vi "Move To Raw Relative.vi"(6 "Rotation Angle":dbl, 7 "Wait?":bool=TRUE, 8 "error in":errorcluster, 9 "Speed(mm/s)":dbl=5.0, 10 "Delta":refnum<class "Vec3d.lvclass">, 11 "Gantry in":refnum<class "Gantry.lvclass">) -> (0 "error out":errorcluster, 3 "Gantry out":refnum<class "Gantry.lvclass">)   [LabVIEW 2026, in "Gantry.lvclass"]
uses:
  Gantry.lvclass
  Vec3d Class/Vec3d.lvclass
  Gantry.lvclass/Gantry.ctl
  <instrlib>/Aerotech Automation1/Commands/Motion/typedefs/MoveLinear parameters.ctl
  <instrlib>/Aerotech Automation1/Aerotech Automation1.lvlib
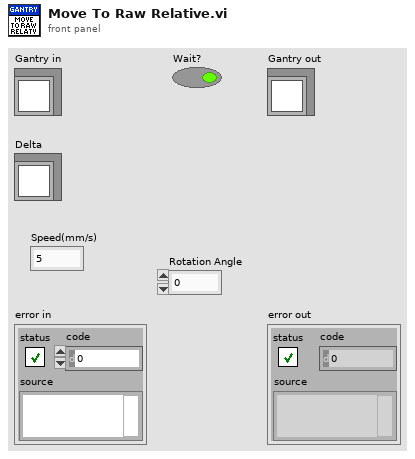
[diagram p1: front panel]
types:
  T1 = typedef "Aerotech Automation1.lvlib/MoveLinear parameters.ctl" = cluster{"coordinatedSpeed":dbl, "distances":dbl[], "axes":string[]}
  T2 = typedef "Virtual Modes.ctl" = enum16{"Nonvirtual", "Virtual"}
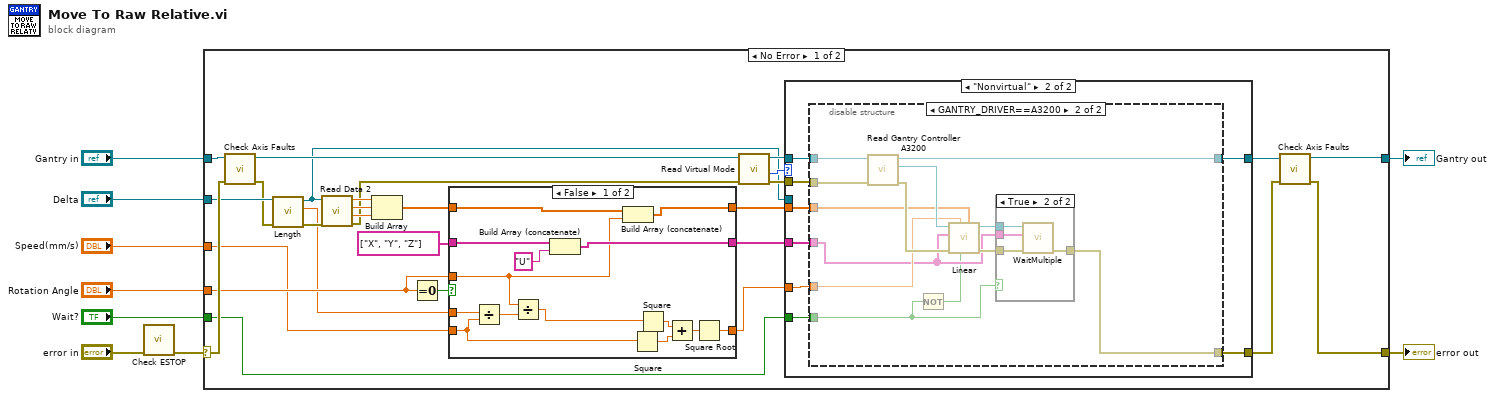
[diagram p0: block diagram]
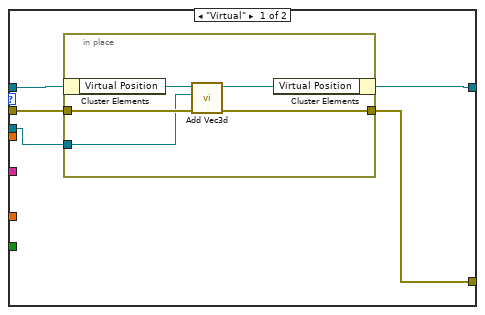
[diagram p3: hidden frame]
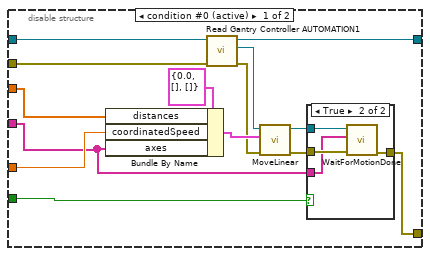
[diagram p4: hidden frame]
diagram:
  n1 = call "Check ESTOP.vi"("error in"="error in") -> ("error out"=w3:errorcluster)  [unwired: 10 in]
  n2 = case shown="No Error" w3 {
    selector: w3 -> [w33 w111]
    tunnel: [w11 w111] -> w8
    tunnel: [w10 w110] -> w7
    tunnel: "Gantry in" -> [w35 w110]
    tunnel: "Speed(mm/s)" -> [w20 _]
    tunnel: "Delta" -> [w18 _]
    tunnel: "Wait?" -> [w28 _]
    tunnel: "Rotation Angle" -> [w24 _]
    frame No Error {
      n3 = call "Check Axis Faults.vi"("error in (no error)"=w33, "Gantry in"=w35) -> ("error out"=w16:errorcluster, "Gantry out"=w34:refnum<class "Gantry.lvclass">)  [unwired: 8 in]
      n4 = call-dynamic "Length.vi"("error in"=w16, "Vec3d in"=w18) -> ("error out"=w15:errorcluster, "Length"=w14:dbl, "Vec3d out"=w17:refnum<class "Vec3d.lvclass">)  [unwired: 7 in]
      n5 = call-dynamic "Read Data 2.vi"("error in"=w15, "Vec3d in"=w17) -> ("error out"=w29:errorcluster, "Z"=w30:dbl, "Y"=w31:dbl, "X"=w32:dbl)  [unwired: 6 in]
      n6 = Build Array(w32, w31, w30) -> (w27:dbl[])
      n7 = Equal To 0?(x=w24) -> (x = 0?=w25:bool)
      n8 = case shown="False" w25 {
        tunnel: w24 -> [w38 _]
        tunnel: w27 -> [w41 w53]
        tunnel: string[] ["X", "Y", "Z"] -> [w43 w52]
        tunnel: w20 -> [w46 w54]
        tunnel: [w48 w54] -> w19
        tunnel: [w40 w53] -> w22
        tunnel: [w39 w52] -> w21
        tunnel: w14 -> [w47 _]
        frame False {
          n9 = Divide(x=w47, y=w46) -> (x/y=w45:dbl)
          n10 = Divide(x=w38, y=w45) -> (x/y=w44:dbl)
          n11 = Build Array (concatenate)(w43, "U") -> (w39:string[])
          n12 = Build Array (concatenate)(w41, w38) -> (w40:dbl[])
          n13 = Square(x=w46) -> (x^2=w51:dbl)
          n14 = Square(x=w44) -> (x^2=w50:dbl)
          n15 = Add(x=w50, y=w51) -> (x+y=w49:dbl)
          n16 = Square Root(x=w49) -> (sqrt(x)=w48:dbl)
        }
        frame True {
        }
      }
      n17 = call-dynamic "Read Virtual Mode.vi"("error in (no error)"=w29, "Gantry in"=w34) -> ("error out"=w23:errorcluster, "Virtual Mode"=w36:T2, "Gantry out"=w37:refnum<class "Gantry.lvclass">)  [unwired: 6 in, 1 out]
      n18 = case shown="\"Nonvirtual\"" w36 {
        tunnel: w28 -> [_ w70]
        tunnel: [w56 w65] -> w12
        tunnel: [w58 w66] -> w13
        tunnel: w37 -> [w59 w72]
        tunnel: w17 -> [w57 _]
        tunnel: w19 -> [_ w71]
        tunnel: w23 -> [w55 w69]
        tunnel: w22 -> [_ w68]
        tunnel: w21 -> [_ w67]
        frame "Virtual" {
          n19 = in-place {
            in-place-border: w55 -> [w62]
            in-place-border: w57 -> [w60]
            in-place-border: [w61] -> w56
            n20 = in-place-cluster #1(w59) -> ("Virtual Position"=w64:refnum<class "Vec3d.lvclass">)
            n21 = call-dynamic "Add Vec3d.vi"("error in (no error)"=w62, 10:"Vec3d Class in"=w60, 11:"Vec3d Class in"=w64) -> ("error out"=w61:errorcluster, "Vec3d Class out"=w63:refnum<class "Vec3d.lvclass">)  [unwired: 7 in]
            n22 = in-place-cluster #1("Virtual Position"=w63) -> (w58:refnum<class "Gantry.lvclass">)
          }
        }
        frame "Nonvirtual" {
          n23 = disable-structure shown="GANTRY_DRIVER==A3200" {
            disable-tunnel: w72 -> [w86 w104]
            disable-tunnel: w69 -> [w85 w103]
            disable-tunnel: w70 -> [w84 w93]
            disable-tunnel: [w74 w96] -> w66
            disable-tunnel: [w75 w95] -> w65
            disable-tunnel: w68 -> [w77 w98]
            disable-tunnel: w71 -> [w76 w99]
            disable-tunnel: w67 -> [w73 w94]
            frame condition #0 (active) {
              n24 = Bundle By Name(cluster=T1 {"coordinatedSpeed"=0.0, "distances"=[], "axes"=[]} ("MoveLinear parameters"), "distances"=w77, "coordinatedSpeed"=w76, "axes"=w73) -> (w83:T1)
              n25 = call "Read Gantry Controller AUTOMATION1.vi"("error in (no error)"=w85, "Gantry in"=w86) -> ("error out"=w80:errorcluster, "Controller AUTOMATION1"=w79:refnum<k24>, "Gantry out"=w74:refnum<class "Gantry.lvclass">)  [unwired: 7 in]
              n26 = call <instrlib>:"MoveLinear.vi"("error in (no error)"=w80, "MoveLinear parameters"=w83, "Controller Refnum"=w79) -> ("error out"=w78:errorcluster, "Controller Refnum out"=w81:refnum<k24>)  [unwired: 7 in]
              n27 = case shown="True" w84 {
                tunnel: w81 -> [_ w91]
                tunnel: w78 -> [w87 w90]
                tunnel: [w87 w89] -> w75
                tunnel: w73 -> [_ w88]
                frame False {
                }
                frame True {
                  n28 = call <instrlib>:"WaitForMotionDone.vi"("error in (no error)"=w90, "axes"=w88, "Controller Refnum"=w91) -> ("error out"=w89:errorcluster)  [unwired: 7 in, 1 out]
                }
              }
            }
            frame condition #1 {
              n29 = call "Read Gantry Controller A3200.vi"("error in (no error)"=w103, "Gantry in"=w104) -> ("error out"=w101:errorcluster, "A3200 controller out"=w102:refnum<k24>, "Gantry out"=w96:refnum<class "Gantry.lvclass">)  [unwired: 7 in]
              n30 = Not(x=w93) -> (.not. x?=w92:bool)
              n31 = call "Linear.vi"("distances"=w98, "return immediately"=w92, "speed"=w99, "error in (no error)"=w101, "axis names"=w94, "controller in"=w102) -> ("error out"=w100:errorcluster, "controller out"=w97:refnum<k24>)  [unwired: 4 in]
              n32 = case shown="True" w93 {
                tunnel: w100 -> [w105 w109]
                tunnel: w97 -> [_ w108]
                tunnel: [w105 w107] -> w95
                tunnel: w94 -> [_ w106]
                frame False {
                }
                frame True {
                  n33 = call "WaitMultiple.vi"("error in (no error)"=w109, "axis names"=w106, "controller in"=w108) -> ("error out"=w107:errorcluster)  [unwired: 6 in, 2 out]
                }
              }
            }
          }
        }
      }
      n34 = call "Check Axis Faults.vi"("error in (no error)"=w12, "Gantry in"=w13) -> ("error out"=w11:errorcluster, "Gantry out"=w10:refnum<class "Gantry.lvclass">)  [unwired: 8 in]
    }
    frame Error {
    }
  }
  "error out" <- w8
  "Gantry out" <- w7
